vi "Drive testing.vi"() -> ()   [LabVIEW 2021]
uses:
  Sub VIs/Logging/Controller Data.ctl
  Sub VIs/Drive Motor/Drive Motor Data.ctl
  Sub VIs/Steering Motor/Steering Motor Data.ctl
  <vilib>/Platform/TimedLoop/XDataNode/timing_clust.ctl
  <vilib>/Platform/TimedLoop/XDataNode/nitl_modes.ctl
  <vilib>/Platform/TimedLoop/XDataNode/wakeup.ctl
  <vilib>/Platform/TimedLoop/XDataNode/XDataNode.xnode
  <vilib>/Platform/TimedLoop/XDataNode/XDNodeRunTimeDep.lvlib
panel:
  out "Speed":bool
  in  "?":bool
  out "RPM":bool
  in  "Drive Motor Speed (m/s)":dbl
  in  "Drive Motor Angular Speed (rad/s)":dbl
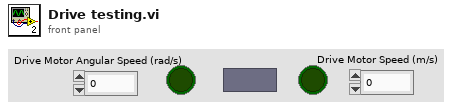
[diagram p1: front panel]
types:
  T1 = typedef "XDNodeRunTimeDep.lvlib/timing_clust.ctl" = cluster{"Expected End [f-1]":u64, "Actual End [f-1]":u64, "Finished Late? [f-1]":bool, "Expected End [i-1]":u64, "Actual End [i-1]":u64, "Finished Late? [i-1]":bool, "Expected Start [i]":u64, "Actual Start [i]":u64, "Expected Start [f]":u64, "Actual Start [f]":u64, "Source Name":string, "Structure Name":string, "Period":i64, "Deadline":i64, "Offset":i64, "Start":i64, "Priority":i32, "Timeout":i32, "Mode":T2, "Wakeup Reason":T3, "Error":errorcluster, "Source Type":string, "Secondary Source Type":string, "Global End Time":u64, "Global Start Time":u64, "Frame Duration":u64, "Iteration Duration":u64, "Assigned CPU":i32, "I/O Scan Engine Mode":u32}
  T2 = typedef "XDNodeRunTimeDep.lvlib/nitl_modes.ctl" = enum32{"No Change", "Process missed periods, maintain original phase", "Discard missed periods, maintain original phase", "Process missed periods, ignore original phase", "Discard missed periods, ignore original phase"}
  T3 = typedef "XDNodeRunTimeDep.lvlib/wakeup.ctl" = enum32{"Normal", "Aborted", "Asynchronous wakeup", "Timing source error", "Timed loop error", "Timeout"}
  T4 = typedef "Drive Motor Handle.ctl" = cluster{"VISA Resource Name":refnum<visa-resource-name>}
  T5 = typedef "Controller Data.ctl" = cluster{"Drive Motor Data":T6, "Steering Motor Data":T7}
  T6 = typedef "Drive Motor Data.ctl" = cluster{"Angular Speed (rad/s)":dbl, "Input Current (A)":dbl, "Motor Current (A)":dbl, "MOSFET Temperature (deg C)":dbl, "Reference Speed (rad/s)":dbl, "PI Current (A)":dbl, "Ki":dbl, "Kp":dbl}
  T7 = typedef "Steering Motor Data.ctl" = cluster{"PWM":dbl, "Steering Angle Rate (rad/s)":dbl, "input balancing":dbl}
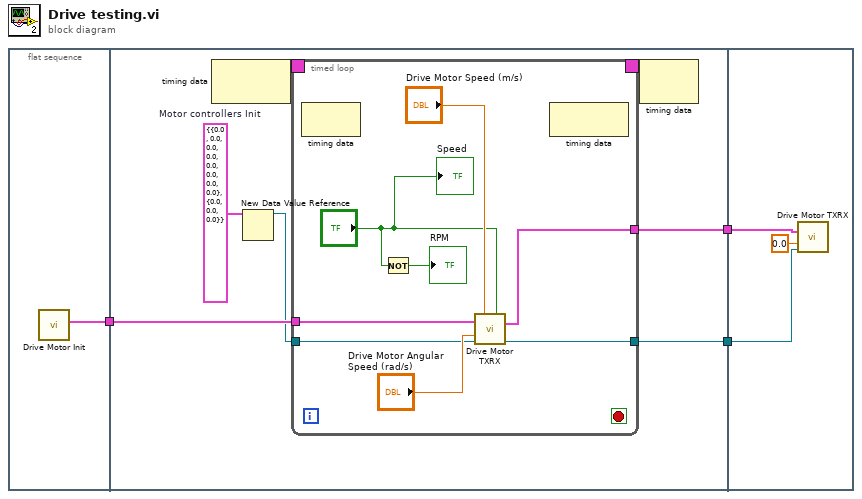
[diagram p0: block diagram]
diagram:
  n1 = flat-sequence {
    tunnel: [w4] -> w3
    tunnel: w3 -> [w11]
    tunnel: [w6] -> w2
    tunnel: [w5] -> w1
    tunnel: w2 -> [w25]
    tunnel: w1 -> [w24]
    frame #0 {
      n2 = call "Drive Motor Init.vi"() -> ("Drive Motor Handle"=w4:T4)  [unwired: 10 in, 1 out]
    }
    frame #1 {
      w8 = T5 {"Drive Motor Data"={"Angular Speed (rad/s)"=0.0, "Input Current (A)"=0.0, "Motor Current (A)"=0.0, "MOSFET Temperature (deg C)"=0.0, "Reference Speed (rad/s)"=0.0, "PI Current (A)"=0.0, "Ki"=0.0, "Kp"=0.0}, "Steering Motor Data"={"PWM"=0.0, "Steering Angle Rate (rad/s)"=0.0, "input balancing"=0.0}}  # Motor controllers Init
      n3 = node-c288() -> (w10:T1)  [unwired: 1 in]
      n4 = New Data Value Reference(data value=w8) -> (data value reference=w7:refnum<data-value>)  [unwired: 1 in, 1 out]
      n5 = timed-loop {
        timing: w10 -> [_]
        timing-out: [_] -> w9
        tunnel: w11 -> [w15]
        tunnel: w7 -> [w14]
        tunnel: [w13] -> w6
        tunnel: [w12] -> w5
        stop <- _ stop-if-true
        n6 = node-c288() -> ()  [unwired: 1 in, 1 out]
        n7 = Not(x="?") -> (.not. x?=→"RPM":bool)
        n8 = call "Drive Motor TXRX.vi"("Speed Control (m/s)"="Drive Motor Speed (m/s)", "RPM / Speed"="?", "Drive Motor Handle In"=w15, "RPM Control (rad/s)"="Drive Motor Angular Speed (rad/s)", "Controller Data In"=w14) -> ("Drive Motor Handle Out"=w12:T4, "Controller Data Out"=w13:refnum<data-value>)  [unwired: 7 in, 2 out]
        n9 = node-c288() -> ()  [unwired: 1 in, 1 out]
        "Speed" <- "?"
      }
      n10 = node-c288(w9) -> ()  [unwired: 1 out]
    }
    frame #2 {
      n11 = call "Drive Motor TXRX.vi"("Drive Motor Handle In"=w24, "RPM Control (rad/s)"=0.0, "Controller Data In"=w25) -> ()  [unwired: 9 in, 4 out]
    }
  }
